vi "Local Transition Outward.vi"(8 "error in (no error)":errorcluster, 10 "Timeout Period in ms (-1, never)":i32=-1, 11 "State Machine Actor in":refnum<class "State Machine Actor.lvclass">) -> (0 "error out":errorcluster, 3 "State Machine Actor out":refnum<class "State Machine Actor.lvclass">)   [LabVIEW 2024, in "State Machine Actor.lvlib" / "State Machine Actor.lvclass"]
uses:
  State Machine Actor.lvclass
  State Machine Actor.lvclass/State Machine Actor.ctl
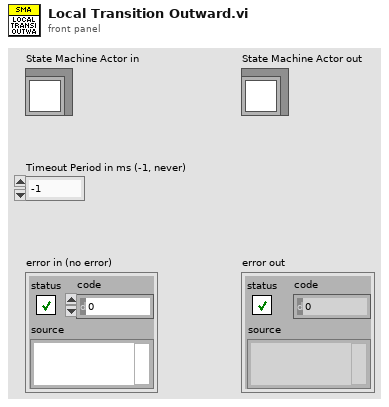
[diagram p1: front panel]
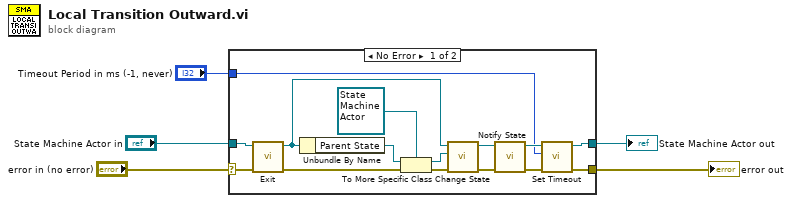
[diagram p0: block diagram]
diagram:
  n1 = case shown="No Error" "error in (no error)" {
    selector: "error in (no error)" -> [w20 w22]
    tunnel: "State Machine Actor in" -> [w7 w21]
    tunnel: "Timeout Period in ms (-1, never)" -> [w16 _]
    tunnel: [w13 w22] -> w4
    tunnel: [w17 w21] -> w1
    frame No Error {
      n2 = call-dynamic "Exit.vi"("error in (no error)"=w20, "State Machine Actor in"=w7) -> ("error out"=w9:errorcluster, "State Machine Actor out"=w11:refnum<class "State Machine Actor.lvclass">)  [unwired: 8 in]
      n3 = Unbundle By Name(w11) -> ("Parent State"=w12:refnum<class "_State Machine Actor.lvclass">)
      n4 = To More Specific Class(target class=refnum<class "State Machine Actor.lvclass"> refnum ("State Machine Actor.lvlib:State Machine Actor.lvclass"), reference=w12, error in=w9) -> (specific class reference=w10:refnum<class "State Machine Actor.lvclass">, error out=w8:errorcluster)
      n5 = call-dynamic "Change State.vi"("error in (no error)"=w8, "Target State"=w10, "State Machine Actor in"=w11) -> ("error out"=w14:errorcluster, "State Machine Actor out"=w19:refnum<class "State Machine Actor.lvclass">)  [unwired: 7 in]
      n6 = call-dynamic "Notify State.vi"("error in (no error)"=w14, "State Machine Actor in"=w19) -> ("error out"=w15:errorcluster, "State Machine Actor out"=w18:refnum<class "State Machine Actor.lvclass">)  [unwired: 8 in]
      n7 = call-dynamic "Set Timeout.vi"("error in (no error)"=w15, "Timeout Period in ms (-1, never)"=w16, "State Machine Actor in"=w18) -> ("error out"=w13:errorcluster, "State Machine Actor out"=w17:refnum<class "State Machine Actor.lvclass">)  [unwired: 7 in]
    }
    frame Error {
    }
  }
  "error out" <- w4
  "State Machine Actor out" <- w1
